vi "JSON Flatten Configuration.vi"(8 "error in (no error)":errorcluster, 10 "file version":T1, 11 "configuration":T2={"custom settings"=[], "plugins"=[{"core settings"={"component"="Plugin", "values"=[]}, "component settings"=[], "threads"=[]}]}) -> (0 "error out":errorcluster, 2 "actual file version":T1, 3 "configuration json":string)   [LabVIEW 2017, in "DSF Core.lvlib" / "Configuration Session.lvclass"]
uses:
  Configuration Session.lvclass
  Typedefs/DSF Engine Framework Configuration.ctl
  Typedefs/DSF Settings Info.ctl
  Typedefs/DSF Engine Plugin Configuration.ctl
  Typedefs/DSF Engine Plugin Thread Configuration.ctl
  Typedefs/DSF Engine Transfer Group Configuration.ctl
  Typedefs/DSF Engine Transfer Configuration.ctl
  Typedefs/DSF Engine Channel Configuration.ctl
  Typedefs/DSF Version Info.ctl
  DSF Core.lvlib
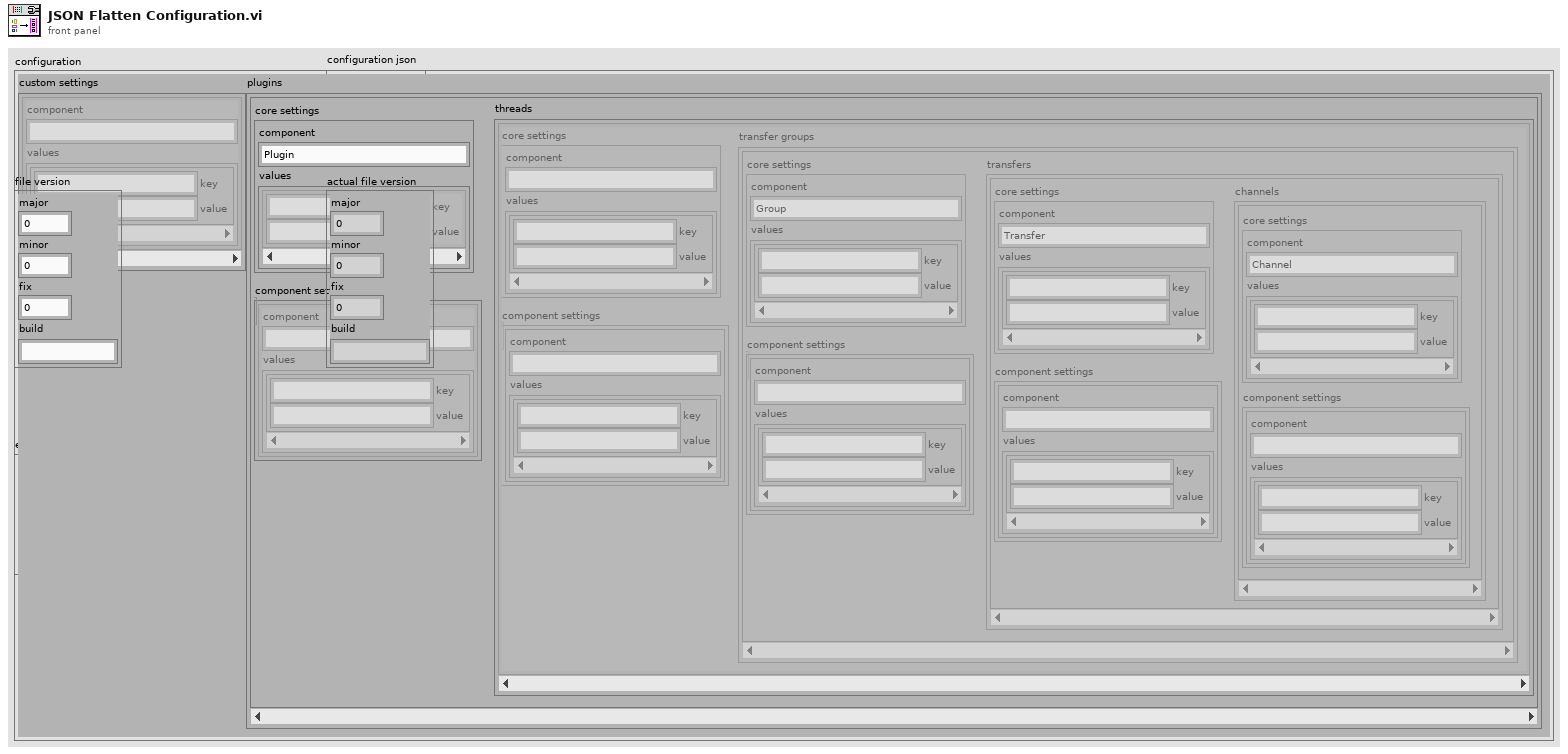
[diagram p1: front panel]
types:
  T1 = typedef "DSF Core.lvlib/DSF Version Info.ctl" = cluster{"major":u32, "minor":u32, "fix":u32, "build":string}
  T2 = typedef "DSF Core.lvlib/DSF Engine Framework Configuration.ctl" = cluster{"custom settings":T3[], "plugins":T4[]}
  T3 = typedef "DSF Core.lvlib/DSF Settings Info.ctl" = cluster{"component":string, "values":cluster{"key":string, "value":string}[]}
  T4 = typedef "DSF Core.lvlib/DSF Engine Plugin Configuration.ctl" = cluster{"core settings":T3, "component settings":T3[], "threads":T5[]}
  T5 = typedef "DSF Core.lvlib/DSF Engine Plugin Thread Configuration.ctl" = cluster{"core settings":T3, "component settings":T3[], "transfer groups":T6[]}
  T6 = typedef "DSF Core.lvlib/DSF Engine Transfer Group Configuration.ctl" = cluster{"core settings":T3, "component settings":T3[], "transfers":T7[]}
  T7 = typedef "DSF Core.lvlib/DSF Engine Transfer Configuration.ctl" = cluster{"core settings":T3, "component settings":T3[], "channels":T8[]}
  T8 = typedef "DSF Core.lvlib/DSF Engine Channel Configuration.ctl" = cluster{"core settings":T3, "component settings":T3[]}
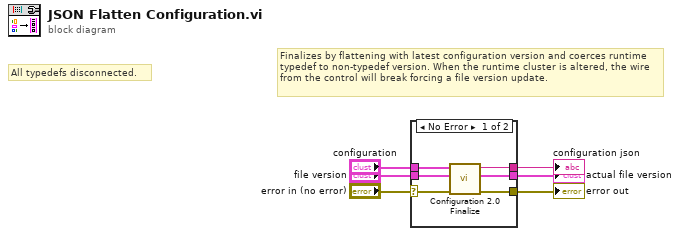
[diagram p0: block diagram]
diagram:
  # "Finalizes by flattening with latest configuration version and coerces runtime typedef to non-typedef version. When the runtime cluster is altered, the wire from the control will break forcing a file version update."
  # "All typedefs disconnected."
  n1 = case shown="No Error" "error in (no error)" {
    selector: "error in (no error)" -> [w12 w13]
    tunnel: [w7 w13] -> w6
    tunnel: [w9 _] -> w4
    tunnel: [w8 _] -> w3
    tunnel: "file version" -> [w10 _]
    tunnel: "configuration" -> [w11 _]
    frame No Error {
      n2 = call "Configuration 2.0 Finalize.vi"("error in (no error)"=w12, "file version (2.0)"=w10, "configuration 2.0"=w11) -> ("error out"=w7:errorcluster, "final file version"=w8:T1, "configuration json"=w9:string)  [unwired: 6 in]
    }
    frame Error {
    }
  }
  "configuration json" <- w4
  "error out" <- w6
  "actual file version" <- w3
